vi "Launch SCADA.vi"(8 "error in (no error)":errorcluster, 11 "Master Controller in":refnum<class "Master Controller.lvclass">) -> (0 "error out":errorcluster, 3 "Master Controller out":refnum<class "Master Controller.lvclass">)   [LabVIEW 2015, in "Master Controller Core.lvlib" / "Master Controller.lvclass"]
uses:
  Master Controller.lvclass
  SCADA Core/SCADA/SCADA.lvclass
  SCADA Core/SCADA/Controls/Abstract Messages Definitions Cluster.ctl
  SCADA Core/SCADA Abstract Messages/Simple Command Status Msg/Simple Command Status Msg.lvclass
  SCADA Core/SCADA Abstract Messages/Black Start Status Msg/Black Start Status Msg.lvclass
  SCADA Core/SCADA Abstract Messages/IED Measurement Status Msg/IED Measurement Status Msg.lvclass
  SCADA Core/SCADA Abstract Messages/Device Action Status Msg/Device Action Status Msg.lvclass
  SCADA Core/SCADA Abstract Messages/Device Load Status Msg/Device Load Status Msg.lvclass
  SCADA Core/SCADA Abstract Messages/IED Setpoint Status Msg/IED Setpoint Status Msg.lvclass
  SCADA Core/SCADA Abstract Messages/Get Device Parameter Status Msg/Get Device Parameter Status Msg.lvclass
  SCADA Core/SCADA Abstract Messages/Set Device Parameter Status Msg/Set Device Parameter Status Msg.lvclass
  SCADA Core/SCADA Abstract Messages/Set Shed Sequence Status Msg/Set Shed Sequence Status Msg.lvclass
  SCADA Core/SCADA Abstract Messages/Emergency Status Msg/Emergency Status Msg.lvclass
  Master Controller Messages/EMS Activate Status Msg/EMS Activate Status Msg.lvclass
  Master Controller Messages/EMS Shutdown Status Msg/EMS Shutdown Status Msg.lvclass
  Master Controller Messages/EMS Island Control Status Msg/EMS Island Control Status Msg.lvclass
  Master Controller Messages/EMS PCC Relay Status Msg/EMS PCC Relay Status Msg.lvclass
  Master Controller Messages/EMS Device Load Status Msg/EMS Device Load Status Msg.lvclass
  Master Controller Messages/EMS Device Unload Status Msg/EMS Device Unload Status Msg.lvclass
  Master Controller Messages/EMS Setpoint Status Msg/EMS Setpoint Status Msg.lvclass
  Master Controller Messages/EMS Get Device Parameter Status Msg/EMS Get Device Parameter Status Msg.lvclass
  Master Controller Messages/EMS Set Device Parameter Status Msg/EMS Set Device Parameter Status Msg.lvclass
  Master Controller Messages/EMS Get Measurement Status Msg/EMS Get Measurement Status Msg.lvclass
  Master Controller Messages/Notify Device Activate Failure Msg/Notify Device Activate Failure Msg.lvclass
  Master Controller Messages/Notify Islanded Msg/Notify Islanded Msg.lvclass
  Master Controller Messages/Notify Fatal Error Msg/Notify Fatal Error Msg.lvclass
  Master Controller Messages/EMS Black Start Status Msg/EMS Black Start Status Msg.lvclass
  Master Controller Messages/EMS Set Shed Sequence Status Msg/EMS Set Shed Sequence Status Msg.lvclass
  Master Controller Messages/EMS Device Activate Status Msg/EMS Device Activate Status Msg.lvclass
  Master Controller Messages/EMS Synchronize Status Msg/EMS Synchronize Status Msg.lvclass
  Master Controller Messages/EMS Island Status Msg/EMS Island Status Msg.lvclass
  Master Controller Messages/EMS Measurement Visualization Msg/EMS Measurement Visualization Msg.lvclass
  Master Controller.lvclass/Master Controller.ctl
  SCADA Core/SCADA/SCADA.lvclass/SCADA.ctl
  <vilib>/ActorFramework/Actor/Actor.lvclass
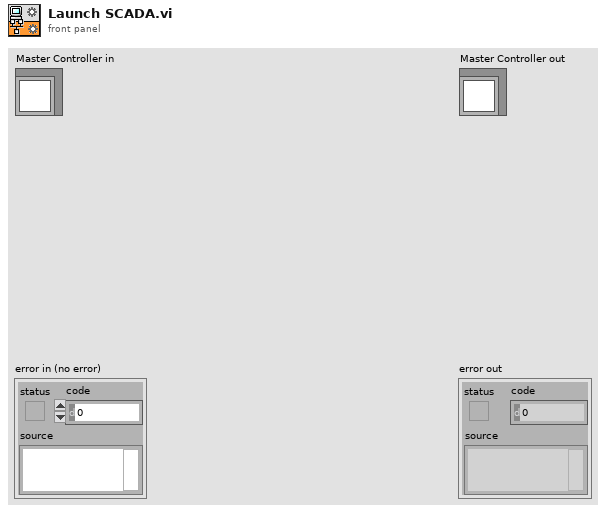
[diagram p1: front panel]
types:
  T1 = typedef "SCADA Core.lvlib/SCADA.lvclass/Abstract Messages Definitions Cluster.ctl" = cluster{"Activate Status Msg":refnum<class "Simple Command Status Msg.lvclass">, "Black Start Status Msg":refnum<class "Black Start Status Msg.lvclass">, "Shutdown Status Msg":refnum<class "Simple Command Status Msg.lvclass">, "Synchronize Status Msg":refnum<class "Simple Command Status Msg.lvclass">, "Island Status Msg":refnum<class "Simple Command Status Msg.lvclass">, "IED Measurement Msg":refnum<class "IED Measurement Status Msg.lvclass">, "Device Activate Status Msg":refnum<class "Device Action Status Msg.lvclass">, "Island Control Status Msg":refnum<class "Device Action Status Msg.lvclass">, "PCC Relay Status Msg":refnum<class "Device Action Status Msg.lvclass">, "Device Load Status Msg":refnum<class "Device Load Status Msg.lvclass">, "Device Unload Status Msg":refnum<class "Device Action Status Msg.lvclass">, "IED Setpoint Status Msg":refnum<class "IED Setpoint Status Msg.lvclass">, "Get Device Parameter Status Msg":refnum<class "Get Device Parameter Status Msg.lvclass">, "Set Device Parameter Status Msg":refnum<class "Set Device Parameter Status Msg.lvclass">, "Set Shed Sequence Status Msg":refnum<class "Set Shed Sequence Status Msg.lvclass">, "Device Activate Failure Msg":refnum<class "Emergency Status Msg.lvclass">, "Islanded Msg":refnum<class "Emergency Status Msg.lvclass">, "Fatal Error Msg":refnum<class "Emergency Status Msg.lvclass">, "Measurement Visualization Msg":refnum<class "IED Measurement Status Msg.lvclass">}
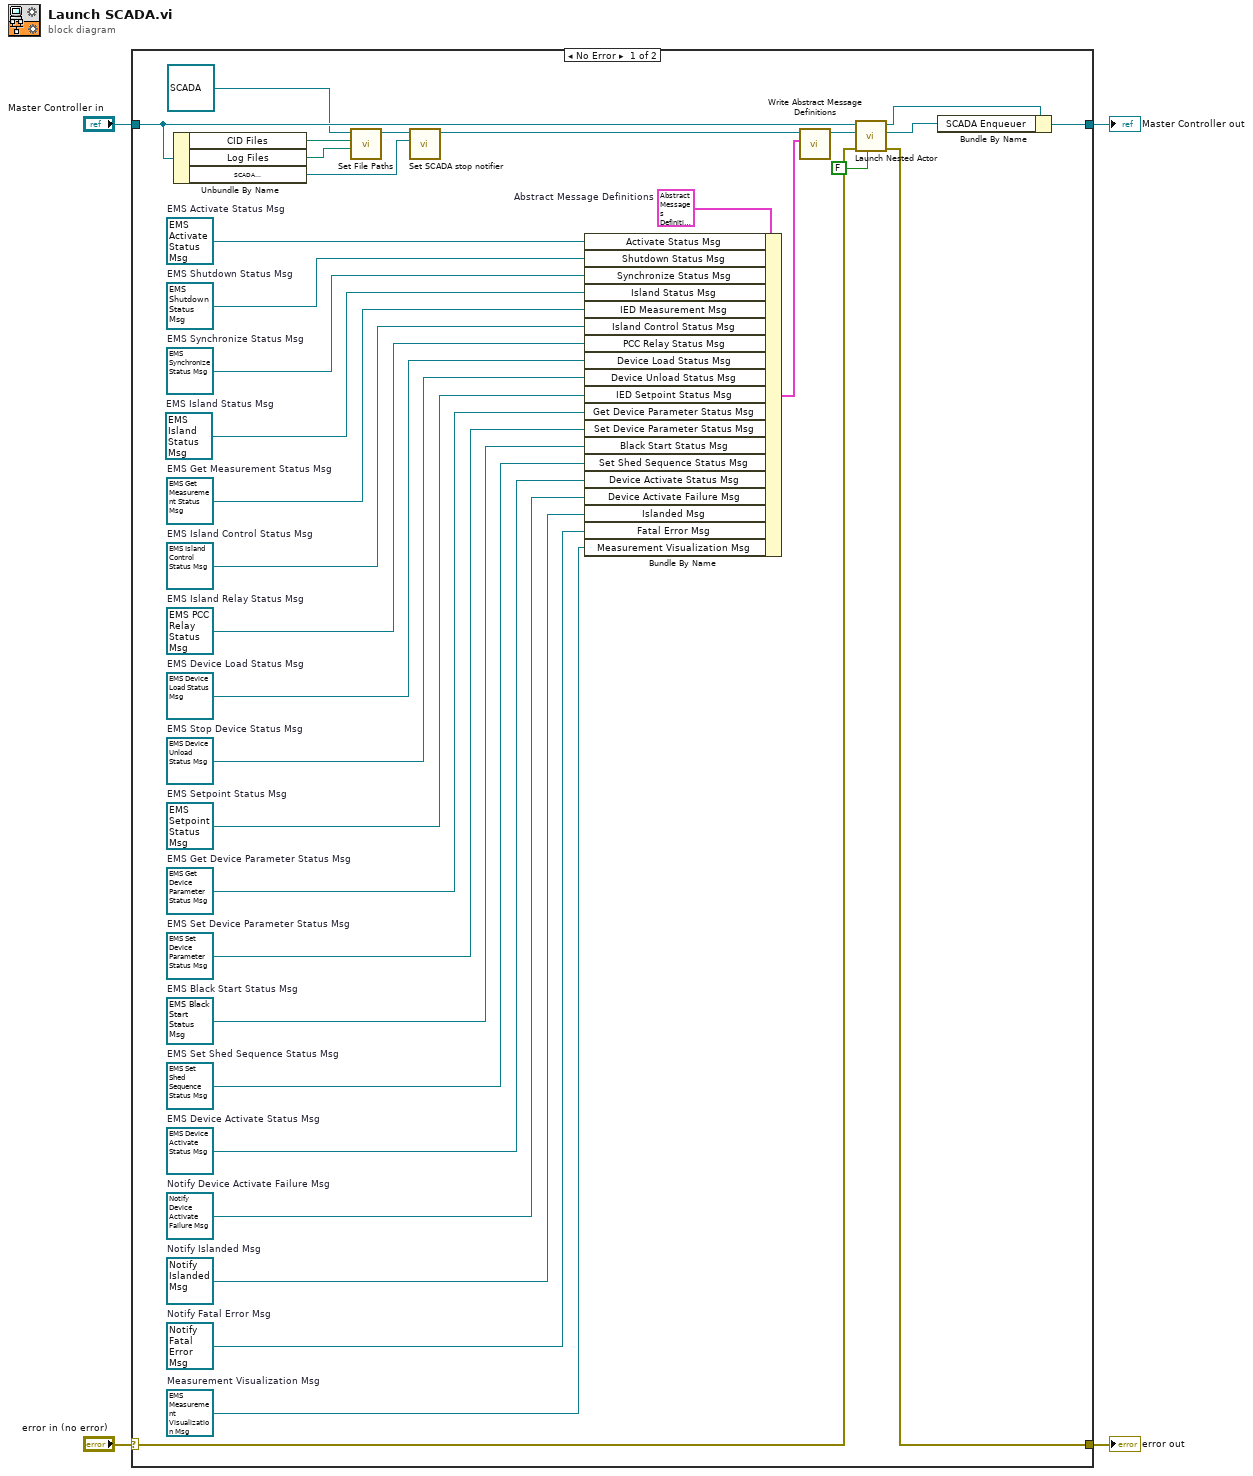
[diagram p0: block diagram]
diagram:
  n1 = case shown="No Error" "error in (no error)" {
    selector: "error in (no error)" -> [w35 w41]
    tunnel: [w36 w41] -> w3
    tunnel: [w38 w40] -> w1
    tunnel: "Master Controller in" -> [w31 w40]
    frame No Error {
      w9 = refnum<class "EMS Measurement Visualization Msg.lvclass"> refnum  # Measurement Visualization Msg
      w10 = refnum<class "EMS Island Status Msg.lvclass"> refnum  # EMS Island Status Msg
      w11 = refnum<class "EMS Synchronize Status Msg.lvclass"> refnum  # EMS Synchronize Status Msg
      w13 = refnum<class "EMS Device Activate Status Msg.lvclass"> refnum  # EMS Device Activate Status Msg
      w17 = refnum<class "EMS Set Shed Sequence Status Msg.lvclass"> refnum  # EMS Set Shed Sequence Status Msg
      w18 = refnum<class "EMS Black Start Status Msg.lvclass"> refnum  # EMS Black Start Status Msg
      w14 = refnum<class "Notify Fatal Error Msg.lvclass"> refnum  # Notify Fatal Error Msg
      w15 = refnum<class "Notify Islanded Msg.lvclass"> refnum  # Notify Islanded Msg
      w16 = refnum<class "Notify Device Activate Failure Msg.lvclass"> refnum  # Notify Device Activate Failure Msg
      w26 = refnum<class "EMS Get Measurement Status Msg.lvclass"> refnum  # EMS Get Measurement Status Msg
      w19 = refnum<class "EMS Set Device Parameter Status Msg.lvclass"> refnum  # EMS Set Device Parameter Status Msg
      w20 = refnum<class "EMS Get Device Parameter Status Msg.lvclass"> refnum  # EMS Get Device Parameter Status Msg
      w21 = refnum<class "EMS Setpoint Status Msg.lvclass"> refnum  # EMS Setpoint Status Msg
      w22 = refnum<class "EMS Device Unload Status Msg.lvclass"> refnum  # EMS Stop Device Status Msg
      w23 = refnum<class "EMS Device Load Status Msg.lvclass"> refnum  # EMS Device Load Status Msg
      w24 = refnum<class "EMS PCC Relay Status Msg.lvclass"> refnum  # EMS Island Relay Status Msg
      w25 = refnum<class "EMS Island Control Status Msg.lvclass"> refnum  # EMS Island Control Status Msg
      w27 = refnum<class "EMS Shutdown Status Msg.lvclass"> refnum  # EMS Shutdown Status Msg
      w28 = refnum<class "EMS Activate Status Msg.lvclass"> refnum  # EMS Activate Status Msg
      w33 = T1 {"Activate Status Msg"=refnum, "Black Start Status Msg"=refnum, "Shutdown Status Msg"=refnum, "Synchronize Status Msg"=refnum, "Island Status Msg"=refnum, "IED Measurement Msg"=refnum, "Device Activate Status Msg"=refnum, "Island Control Status Msg"=refnum, "PCC Relay Status Msg"=refnum, "Device Load Status Msg"=refnum, "Device Unload Status Msg"=refnum, "IED Setpoint Status Msg"=refnum, "Get Device Parameter Status Msg"=refnum, "Set Device Parameter Status Msg"=refnum, "Set Shed Sequence Status Msg"=refnum, "Device Activate Failure Msg"=refnum, "Islanded Msg"=refnum, "Fatal Error Msg"=refnum, "Measurement Visualization Msg"=refnum}  # Abstract Message Definitions
      n2 = Unbundle By Name(w31) -> ("CID Files"=w29:path, "Log Files"=w12:path, "SCADA\nstop"=w6:refnum<notifier>)
      n3 = call "Set File Paths.vi"("Log File Path"=w12, "CID File Path"=w29, "SCADA in"=refnum<class "SCADA.lvclass"> refnum ("SCADA Core.lvlib:SCADA.lvclass")) -> ("SCADA out"=w8:refnum<class "SCADA.lvclass">)  [unwired: 8 in]
      n4 = call "Set SCADA stop notifier.vi"("SCADA stop"=w6, "SCADA in"=w8) -> ("SCADA out"=w7:refnum<class "SCADA.lvclass">)  [unwired: 9 in]
      n5 = Bundle By Name(cluster=w33, "Activate Status Msg"=w28, "Shutdown Status Msg"=w27, "Synchronize Status Msg"=w11, "Island Status Msg"=w10, "IED Measurement Msg"=w26, "Island Control Status Msg"=w25, "PCC Relay Status Msg"=w24, "Device Load Status Msg"=w23, "Device Unload Status Msg"=w22, "IED Setpoint Status Msg"=w21, "Get Device Parameter Status Msg"=w20, "Set Device Parameter Status Msg"=w19, "Black Start Status Msg"=w18, "Set Shed Sequence Status Msg"=w17, "Device Activate Status Msg"=w13, "Device Activate Failure Msg"=w16, "Islanded Msg"=w15, "Fatal Error Msg"=w14, "Measurement Visualization Msg"=w9) -> (w32:T1)
      n6 = call "Write Abstract Message Definitions.vi"("Abstract Message Definitions"=w32, "SCADA in"=w7) -> ("SCADA out"=w34:refnum<class "SCADA.lvclass">)  [unwired: 9 in]
      n7 = call <vilib>:"Launch Nested Actor.vi"("Open Actor Core front panel? (F)"=FALSE, "error in (no error)"=w35, "Nested Actor"=w34, "Caller Actor in"=w31) -> ("error out"=w36:errorcluster, "Nested Actor's Enqueuer"=w37:refnum<class "Message Enqueuer.lvclass">, "Caller Actor out"=w39:refnum<class "Master Controller.lvclass">)  [unwired: 5 in]
      n8 = Bundle By Name(cluster=w39, "SCADA Enqueuer"=w37) -> (w38:refnum<class "Master Controller.lvclass">)
    }
    frame Error {
    }
  }
  "error out" <- w3
  "Master Controller out" <- w1
